vi "S2C_M2p5942_Proc_CacheState.vi"(7 "Label":string, 8 "Error In":errorcluster, 11 "Data In":string) -> (0 "Error Out":errorcluster, 3 "Data Out":string)   [LabVIEW 2024]
uses:
  S2C_M2p5942_Proc_Globals.vi
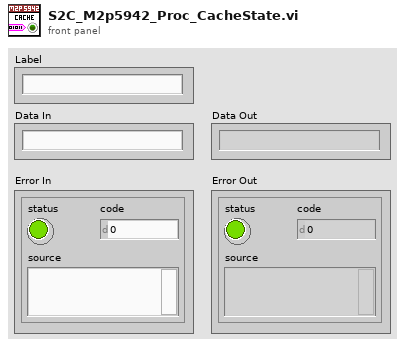
[diagram p1: front panel]
types:
  T1 = cluster{"Index":u32, "IP Address":string, "Device":u16, "P1C1Exe":bool}
  T2 = cluster{"Index":u32, "IP Address":string, "Device":u16}
  T3 = cluster{"CH0 Enable":bool, "CH0 Range":u16, "CH0 Term":u16, "CH0 Type":u16, "CH0 Offset":i32, "CH1 Enable":bool, "CH1 Range":u16, "CH1 Term":u16, "CH1 Type":u16, "CH1 Offset":i32, "CH2 Enable":bool, "CH2 Range":u16, "CH2 Term":u16, "CH2 Type":u16, "CH2 Offset":i32, "CH3 Enable":bool, "CH3 Range":u16, "CH3 Term":u16, "CH3 Type":u16, "CH3 Offset":i32}
  T4 = cluster{"CH1":cluster{"CH0 Enable":bool, "CH0 Range":u16, "CH0 Term":u16, "CH0 Type":u16, "CH0 Offset":i32}, "CH2":cluster{"CH1 Enable":bool, "CH1 Range":u16, "CH1 Term":u16, "CH1 Type":u16, "CH1 Offset":i32}, "CH3":cluster{"CH2 Enable":bool, "CH2 Range":u16, "CH2 Term":u16, "CH2 Type":u16, "CH2 Offset":i32}, "CH4":cluster{"CH3 Enable":bool, "CH3 Range":u16, "CH3 Term":u16, "CH3 Type":u16, "CH3 Offset":i32}, "P2C1Exe":bool}
  T5 = cluster{"Mode":u16, "Memory":u32, "Segment Size":u32, "PostTrigger":u32, "PreTrigger":u32, "ABA Mode":u32, "P2C2Exe":bool}
  T6 = cluster{"Mode":u16, "Memory":u32, "Segment Size":u32, "PostTrigger":u32, "PreTrigger":u32, "ABA Mode":u32}
  T7 = cluster{"Trigger Source":u16, "External Trigger":u16, "EXT Trig Level 0":i32, "EXT Trig Term":bool, "Channel Trigger":u16, "CH Trig Level 0":i32, "CH Trig Level 1":i32, "Trigger Delay":u32, "P3C1Exe":bool}
  T8 = cluster{"Trigger Source":u16, "External Trigger":u16, "EXT Trig Level 0":i32, "EXT Trig Term":bool, "Channel Trigger":u16, "CH Trig Level 0":i32, "CH Trig Level 1":i32, "Trigger Delay":u32}
  T9 = cluster{"Clock Mode":u16, "Sampling Rate (kHz)":dbl, "Clock Output":bool, "Termination":bool, "Ref. Clock (MHz)":dbl, "Threshold (mV)":i32, "P3C2Exe":bool}
  T10 = cluster{"Clock Mode":u16, "Sampling Rate (kHz)":dbl, "Clock Output":bool, "Termination":bool, "Ref. Clock (MHz)":dbl, "Threshold (mV)":i32}
  T11 = cluster{"X0 Mode":u16, "X1 Mode":u16, "X2 Mode":u16, "X3 Mode":u16, "X0 Send":bool, "X1 Send":bool, "X2 Send":bool, "X3 Send":bool, "X1 Trigger Mode":u16, "X2 Trigger Mode":u16, "X3 Trigger Mode":u16, "X1 Pulsewidth":u32, "X2 Pulsewidth":u32, "X3 Pulsewidth":u32, "ASync Read":bool, "ASync Data":i32}
  T12 = cluster{"CH0 Enable":bool, "CH0 Range":u16, "CH0 Term":u16, "CH0 Type":u16, "CH0 Offset":i32}
  T13 = cluster{"CH1 Enable":bool, "CH1 Range":u16, "CH1 Term":u16, "CH1 Type":u16, "CH1 Offset":i32}
  T14 = cluster{"CH2 Enable":bool, "CH2 Range":u16, "CH2 Term":u16, "CH2 Type":u16, "CH2 Offset":i32}
  T15 = cluster{"CH3 Enable":bool, "CH3 Range":u16, "CH3 Term":u16, "CH3 Type":u16, "CH3 Offset":i32}
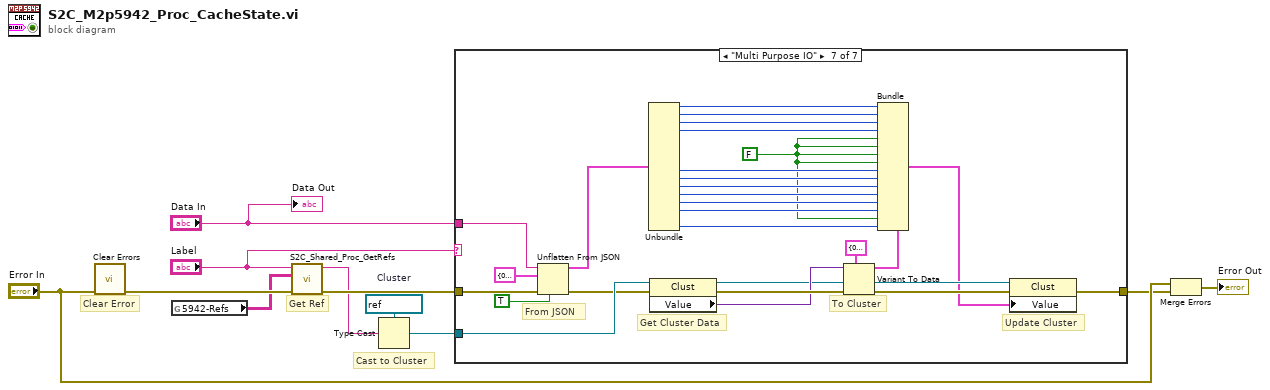
[diagram p0: block diagram]
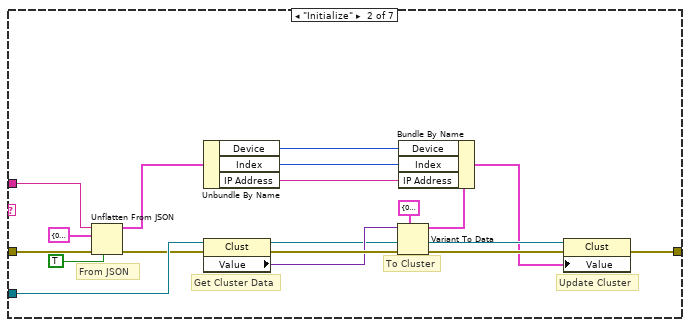
[diagram p3: hidden frame]
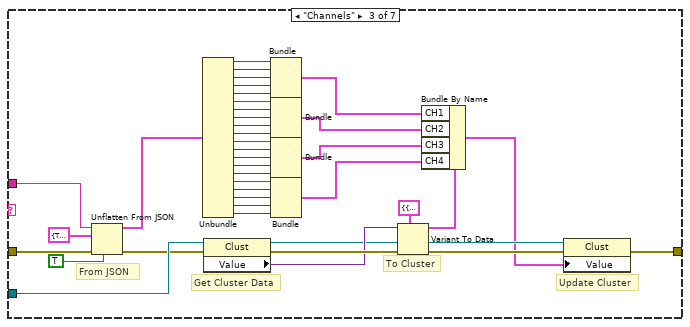
[diagram p4: hidden frame]
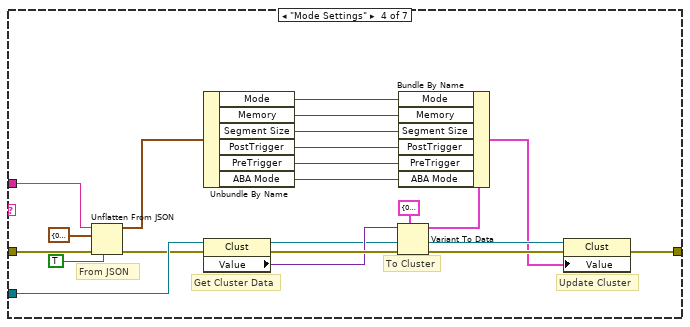
[diagram p5: hidden frame]
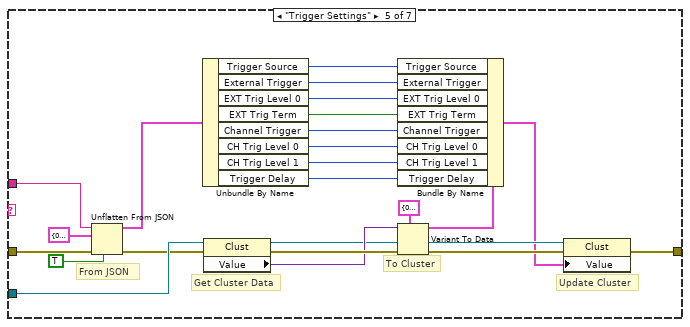
[diagram p6: hidden frame]
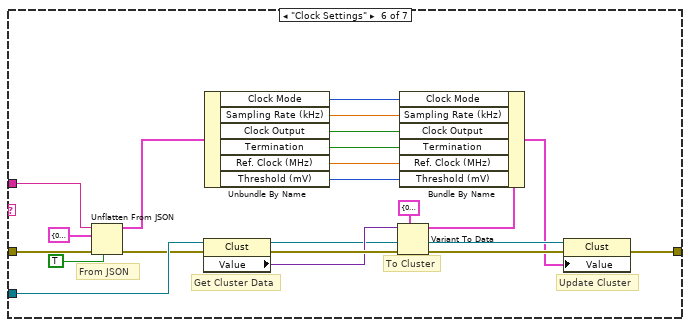
[diagram p7: hidden frame]
diagram:
  w7 = refnum<vi> refnum  # Cluster
  # "Cast to Cluster"
  # "Get Ref"
  # "Clear Error"
  n1 = call <vilib>:"Clear Errors.vi"("error in (no error)"="Error In") -> ("error out"=w4:errorcluster)  [unwired: 5 in, 1 out]
  n2 = global read "S2C_M2p5942_Proc_Globals.vi" "5942-Refs"() -> (w1:string[][])
  n3 = call "S2C_Shared_Proc_GetRefs.vi"("Error In"=w4, "Refs"=w1, "Label"="Label") -> ("Error Out"=w9:errorcluster, "Reference"=w6:string)  [unwired: 7 in]
  n4 = Type Cast(type=w7, x=w6) -> (*(type *) &x=w5:refnum<vi>)
  n5 = case shown="\"Multi Purpose IO\"" "Label" {
    tunnel: w9 -> [w12 w26 w65 w86 w109 w130 w157]
    tunnel: [w12 w22 w61 w82 w105 w126 w153] -> w2
    tunnel: w5 -> [_ w28 w67 w88 w111 w132 w159]
    tunnel: "Data In" -> [_ w25 w64 w85 w108 w129 w156]
    frame "Other", Default {
    }
    frame "Initialize" {
      # "Update Cluster"
      # "To Cluster"
      # "Get Cluster Data"
      # "From JSON"
      n6 = Unflatten From JSON(JSON string=w25, type and defaults=T2 {"Index"=0, "IP Address"="", "Device"=0} ("Initialize"), default null elements? (F)=TRUE, error in (no error)=w26) -> (value=w19:T2, error out=w24:errorcluster)  [unwired: 3 in]
      n7 = Unbundle By Name(w19) -> ("Device"=w14:u16, "Index"=w15:u32, "IP Address"=w16:string)
      n8 = property class="Clust"(reference=w28, error in=w24) -> (reference out=w23:refnum<vi>, error out=w30:errorcluster, "Value"=w29:variant)
      n9 = Variant To Data(error in=w30, type=T1 {"Index"=0, "IP Address"="", "Device"=0, "P1C1Exe"=FALSE} ("Initialize"), Variant=w29) -> (data=w17:T1, error out=w21:errorcluster)
      n10 = Bundle By Name(cluster=w17, "Device"=w14, "Index"=w15, "IP Address"=w16) -> (w13:T1)
      n11 = property class="Clust"(reference=w23, error in=w21, "Value"=w13) -> (error out=w22:errorcluster)  [unwired: 1 out]
    }
    frame "Channels" {
      # "Update Cluster"
      # "To Cluster"
      # "Get Cluster Data"
      # "From JSON"
      n12 = Unflatten From JSON(JSON string=w64, type and defaults=T3 {"CH0 Enable"=TRUE, "CH0 Range"=2, "CH0 Term"=0, "CH0 Type"=0, "CH0 Offset"=0, "CH1 Enable"=TRUE, "CH1 Range"=2, "CH1 Term"=0, "CH1 Type"=0, "CH1 Offset"=0, "CH2 Enable"=TRUE, "CH2 Range"=2, "CH2 Term"=0, "CH2 Type"=0, "CH2 Offset"=0, "CH3 Enable"=TRUE, "CH3 Range"=2, "CH3 Term"=0, "CH3 Type"=0, "CH3 Offset"=0} ("Channels"), default null elements? (F)=TRUE, error in (no error)=w65) -> (value=w59:T3, error out=w63:errorcluster)  [unwired: 3 in]
      n13 = Unbundle(w59) -> ("CH0 Enable"=w55:bool, "CH0 Range"=w51:u16, "CH0 Term"=w52:u16, "CH0 Type"=w53:u16, "CH0 Offset"=w54:i32, "CH1 Enable"=w48:bool, "CH1 Range"=w45:u16, "CH1 Term"=w44:u16, "CH1 Type"=w43:u16, "CH1 Offset"=w42:i32, "CH2 Enable"=w47:bool, "CH2 Range"=w41:u16, "CH2 Term"=w40:u16, "CH2 Type"=w39:u16, "CH2 Offset"=w38:i32, "CH3 Enable"=w46:bool, "CH3 Range"=w37:u16, "CH3 Term"=w36:u16, "CH3 Type"=w35:u16, "CH3 Offset"=w34:i32)
      n14 = property class="Clust"(reference=w67, error in=w63) -> (reference out=w62:refnum<vi>, error out=w69:errorcluster, "Value"=w68:variant)
      n15 = Bundle("CH0 Enable"=w55, "CH0 Range"=w51, "CH0 Term"=w52, "CH0 Type"=w53, "CH0 Offset"=w54) -> (w49:T12)  [unwired: 1 in]
      n16 = Bundle("CH1 Enable"=w48, "CH1 Range"=w45, "CH1 Term"=w44, "CH1 Type"=w43, "CH1 Offset"=w42) -> (w33:T13)  [unwired: 1 in]
      n17 = Bundle("CH2 Enable"=w47, "CH2 Range"=w41, "CH2 Term"=w40, "CH2 Type"=w39, "CH2 Offset"=w38) -> (w32:T14)  [unwired: 1 in]
      n18 = Bundle("CH3 Enable"=w46, "CH3 Range"=w37, "CH3 Term"=w36, "CH3 Type"=w35, "CH3 Offset"=w34) -> (w31:T15)  [unwired: 1 in]
      n19 = Variant To Data(error in=w69, type=T4 {"CH1"={"CH0 Enable"=TRUE, "CH0 Range"=2, "CH0 Term"=0, "CH0 Type"=0, "CH0 Offset"=0}, "CH2"={"CH1 Enable"=TRUE, "CH1 Range"=2, "CH1 Term"=0, "CH1 Type"=0, "CH1 Offset"=0}, "CH3"={"CH2 Enable"=TRUE, "CH2 Range"=2, "CH2 Term"=0, "CH2 Type"=0, "CH2 Offset"=0}, "CH4"={"CH3 Enable"=TRUE, "CH3 Range"=2, "CH3 Term"=0, "CH3 Type"=0, "CH3 Offset"=0}, "P2C1Exe"=FALSE} ("Channels"), Variant=w68) -> (data=w58:T4, error out=w60:errorcluster)
      n20 = Bundle By Name(cluster=w58, "CH1"=w49, "CH2"=w33, "CH3"=w32, "CH4"=w31) -> (w57:T4)
      n21 = property class="Clust"(reference=w62, error in=w60, "Value"=w57) -> (error out=w61:errorcluster)  [unwired: 1 out]
    }
    frame "Mode Settings" {
      # "Update Cluster"
      # "To Cluster"
      # "Get Cluster Data"
      # "From JSON"
      n22 = Unflatten From JSON(JSON string=w85, type and defaults=T6 {"Mode"=0, "Memory"=16384, "Segment Size"=1024, "PostTrigger"=8192, "PreTrigger"=32, "ABA Mode"=16} ("Mode Settings"), default null elements? (F)=TRUE, error in (no error)=w86) -> (value=w80:T6, error out=w84:errorcluster)  [unwired: 3 in]
      n23 = Unbundle By Name(w80) -> ("Mode"=w77:u16, "Memory"=w76:u32, "Segment Size"=w75:u32, "PostTrigger"=w74:u32, "PreTrigger"=w73:u32, "ABA Mode"=w72:u32)
      n24 = property class="Clust"(reference=w88, error in=w84) -> (reference out=w83:refnum<vi>, error out=w90:errorcluster, "Value"=w89:variant)
      n25 = Variant To Data(error in=w90, type=T5 {"Mode"=0, "Memory"=16384, "Segment Size"=1024, "PostTrigger"=8192, "PreTrigger"=32, "ABA Mode"=16, "P2C2Exe"=FALSE} ("Mode Settings"), Variant=w89) -> (data=w79:T5, error out=w81:errorcluster)
      n26 = Bundle By Name(cluster=w79, "Mode"=w77, "Memory"=w76, "Segment Size"=w75, "PostTrigger"=w74, "PreTrigger"=w73, "ABA Mode"=w72) -> (w78:T5)
      n27 = property class="Clust"(reference=w83, error in=w81, "Value"=w78) -> (error out=w82:errorcluster)  [unwired: 1 out]
    }
    frame "Trigger Settings" {
      # "Update Cluster"
      # "To Cluster"
      # "Get Cluster Data"
      # "From JSON"
      n28 = Unflatten From JSON(JSON string=w108, type and defaults=T8 {"Trigger Source"=0, "External Trigger"=0, "EXT Trig Level 0"=1500, "EXT Trig Term"=TRUE, "Channel Trigger"=0, "CH Trig Level 0"=0, "CH Trig Level 1"=0, "Trigger Delay"=0} ("TriggerSettings"), default null elements? (F)=TRUE, error in (no error)=w109) -> (value=w103:T8, error out=w107:errorcluster)  [unwired: 3 in]
      n29 = Unbundle By Name(w103) -> ("Trigger Source"=w98:u16, "External Trigger"=w97:u16, "EXT Trig Level 0"=w96:i32, "EXT Trig Term"=w95:bool, "Channel Trigger"=w94:u16, "CH Trig Level 0"=w93:i32, "CH Trig Level 1"=w92:i32, "Trigger Delay"=w91:u32)
      n30 = property class="Clust"(reference=w111, error in=w107) -> (reference out=w106:refnum<vi>, error out=w113:errorcluster, "Value"=w112:variant)
      n31 = Variant To Data(error in=w113, type=T7 {"Trigger Source"=0, "External Trigger"=0, "EXT Trig Level 0"=1500, "EXT Trig Term"=TRUE, "Channel Trigger"=0, "CH Trig Level 0"=0, "CH Trig Level 1"=0, "Trigger Delay"=0, "P3C1Exe"=FALSE} ("TriggerSettings"), Variant=w112) -> (data=w102:T7, error out=w104:errorcluster)
      n32 = Bundle By Name(cluster=w102, "Trigger Source"=w98, "External Trigger"=w97, "EXT Trig Level 0"=w96, "EXT Trig Term"=w95, "Channel Trigger"=w94, "CH Trig Level 0"=w93, "CH Trig Level 1"=w92, "Trigger Delay"=w91) -> (w101:T7)
      n33 = property class="Clust"(reference=w106, error in=w104, "Value"=w101) -> (error out=w105:errorcluster)  [unwired: 1 out]
    }
    frame "Clock Settings" {
      # "Update Cluster"
      # "To Cluster"
      # "Get Cluster Data"
      # "From JSON"
      n34 = Unflatten From JSON(JSON string=w129, type and defaults=T10 {"Clock Mode"=0, "Sampling Rate (kHz)"=10000.0, "Clock Output"=TRUE, "Termination"=TRUE, "Ref. Clock (MHz)"=10.0, "Threshold (mV)"=1500} ("Clock Settings"), default null elements? (F)=TRUE, error in (no error)=w130) -> (value=w124:T10, error out=w128:errorcluster)  [unwired: 3 in]
      n35 = property class="Clust"(reference=w132, error in=w128) -> (reference out=w127:refnum<vi>, error out=w134:errorcluster, "Value"=w133:variant)
      n36 = Unbundle By Name(w124) -> ("Clock Mode"=w119:u16, "Sampling Rate (kHz)"=w118:dbl, "Clock Output"=w117:bool, "Termination"=w116:bool, "Ref. Clock (MHz)"=w115:dbl, "Threshold (mV)"=w114:i32)
      n37 = Variant To Data(error in=w134, type=T9 {"Clock Mode"=0, "Sampling Rate (kHz)"=10000.0, "Clock Output"=TRUE, "Termination"=TRUE, "Ref. Clock (MHz)"=10.0, "Threshold (mV)"=1500, "P3C2Exe"=FALSE} ("Clock Settings"), Variant=w133) -> (data=w123:T9, error out=w125:errorcluster)
      n38 = Bundle By Name(cluster=w123, "Clock Mode"=w119, "Sampling Rate (kHz)"=w118, "Clock Output"=w117, "Termination"=w116, "Ref. Clock (MHz)"=w115, "Threshold (mV)"=w114) -> (w122:T9)
      n39 = property class="Clust"(reference=w127, error in=w125, "Value"=w122) -> (error out=w126:errorcluster)  [unwired: 1 out]
    }
    frame "Multi Purpose IO" {
      w137 = FALSE
      # "Update Cluster"
      # "To Cluster"
      # "Get Cluster Data"
      # "From JSON"
      n40 = Unflatten From JSON(JSON string=w156, type and defaults=T11 {"X0 Mode"=0, "X1 Mode"=0, "X2 Mode"=0, "X3 Mode"=0, "X0 Send"=FALSE, "X1 Send"=FALSE, "X2 Send"=FALSE, "X3 Send"=FALSE, "X1 Trigger Mode"=0, "X2 Trigger Mode"=0, "X3 Trigger Mode"=0, "X1 Pulsewidth"=0, "X2 Pulsewidth"=0, "X3 Pulsewidth"=0, "ASync Read"=FALSE, "ASync Data"=0} ("Mulit-PurpIO"), default null elements? (F)=TRUE, error in (no error)=w157) -> (value=w151:T11, error out=w155:errorcluster)  [unwired: 3 in]
      n41 = Unbundle(w151) -> ("X0 Mode"=w148:u16, "X1 Mode"=w138:u16, "X2 Mode"=w139:u16, "X3 Mode"=w140:u16, "X1 Trigger Mode"=w141:u16, "X2 Trigger Mode"=w142:u16, "X3 Trigger Mode"=w143:u16, "X1 Pulsewidth"=w144:u32, "X2 Pulsewidth"=w145:u32, "X3 Pulsewidth"=w146:u32, "ASync Data"=w147:i32)  [unwired: 5 out]
      n42 = property class="Clust"(reference=w159, error in=w155) -> (reference out=w154:refnum<vi>, error out=w161:errorcluster, "Value"=w160:variant)
      n43 = Variant To Data(error in=w161, type=T11 {"X0 Mode"=0, "X1 Mode"=0, "X2 Mode"=0, "X3 Mode"=0, "X0 Send"=FALSE, "X1 Send"=FALSE, "X2 Send"=FALSE, "X3 Send"=FALSE, "X1 Trigger Mode"=0, "X2 Trigger Mode"=0, "X3 Trigger Mode"=0, "X1 Pulsewidth"=0, "X2 Pulsewidth"=0, "X3 Pulsewidth"=0, "ASync Read"=FALSE, "ASync Data"=0} ("Mulit-PurpIO"), Variant=w160) -> (data=w150:T11, error out=w152:errorcluster)
      n44 = Bundle(cluster=w150, "X0 Mode"=w148, "X1 Mode"=w138, "X2 Mode"=w139, "X3 Mode"=w140, "X0 Send"=w137, "X1 Send"=w137, "X2 Send"=w137, "X3 Send"=w137, "X1 Trigger Mode"=w141, "X2 Trigger Mode"=w142, "X3 Trigger Mode"=w143, "X1 Pulsewidth"=w144, "X2 Pulsewidth"=w145, "X3 Pulsewidth"=w146, "ASync Read"=w137, "ASync Data"=w147) -> (w149:T11)
      n45 = property class="Clust"(reference=w154, error in=w152, "Value"=w149) -> (error out=w153:errorcluster)  [unwired: 1 out]
    }
  }
  n46 = Merge Errors("Error In", w2) -> (→"Error Out":errorcluster)
  "Data Out" <- "Data In"
